vi "Check for Valid Header Click.vi"(9 "Button":u16, 10 "Coords":T1, 11 "Table Ref":refnum<vi>) -> (1 "Valid Click?":bool, 3 "Column":i32)   [LabVIEW 2020, in "VI Properties Editor.lvlib"]
doc: "Checks whether a mouse click on the table identified by <B>Table Ref</B> is a valid click, based on the other inputs."
uses:
  VI Properties Editor.lvlib
  <vilib>/Utility/miscctls.llb/LVPoint32TypeDef.ctl
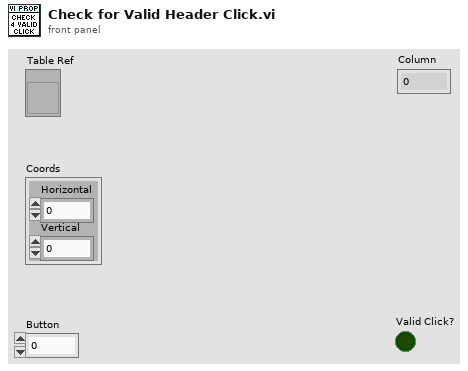
[diagram p1: front panel]
types:
  T1 = typedef "LVPoint32TypeDef.ctl" = cluster{"Horizontal":i32, "Vertical":i32}
  T2 = typedef "LVRowAndColumnTypeDef.ctl" = cluster{"Row":i32, "Column":i32}
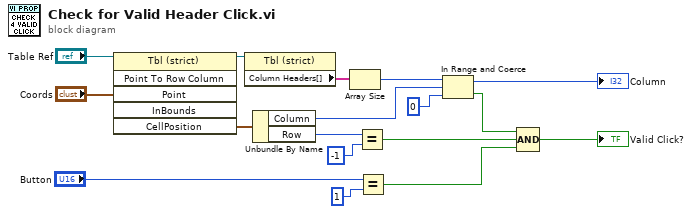
[diagram p0: block diagram]
diagram:
  n1 = invoke on="Invoke Node" class="Tbl (strict)" method="Point To Row Column"(reference="Table Ref", "Point"="Coords") -> (reference out=w17:refnum<vi>, "CellPosition"=w3:T2)  [unwired: 4 in, 4 out]
  n2 = property on="Property Node" class="Tbl (strict)"(reference=w17) -> ("Column Headers[]"=w14:string[])  [unwired: 1 in, 2 out]
  n3 = Unbundle By Name(w3) -> ("Column"=w1:i32, "Row"=w2:i32)
  n4 = Array Size(array=w14) -> (size(s)=w13:i32)
  n5 = Equal?(x=w2, y=-1 ("x")) -> (x = y?=w4:bool)
  n6 = Equal?(x="Button", y=u16 1 ("x")) -> (x = y?=w6:bool)
  n7 = In Range and Coerce(upper limit=w13, x=w1, lower limit=0) -> (coerced(x)=→"Column":i32, In Range?=w12:bool)
  n8 = Compound Arithmetic op=AND(w12, w4, w6) -> (→"Valid Click?":bool)
